vi "New Image.vi"(8 "error in (no error)":errorcluster, 9 "Height":i32, 10 "Width":i32) -> (0 "error out":errorcluster, 3 "Image out":refnum<class "Image.lvclass">)   [LabVIEW 2020, in "RPI.SenseHat.Display.lvlib" / "Image.lvclass"]
uses:
  Image.lvclass
  Pixel/Pixel.lvclass
  Color/Color.lvclass
  Image.lvclass/Image.ctl
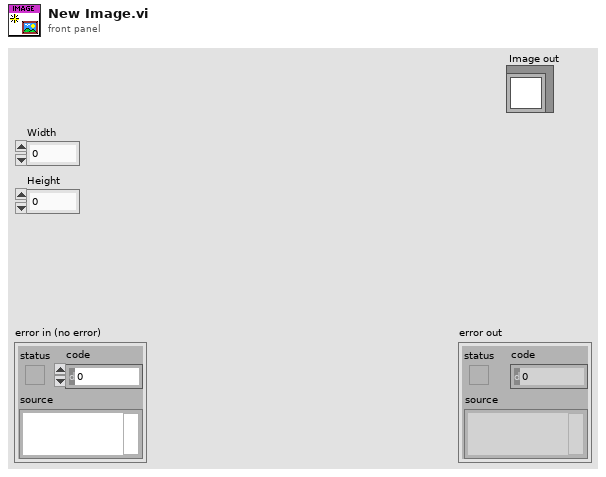
[diagram p1: front panel]
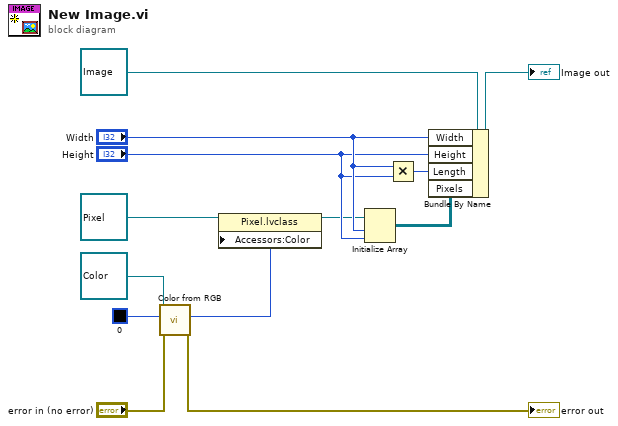
[diagram p0: block diagram]
diagram:
  n1 = call "Color from RGB.vi"("error in (no error)"="error in (no error)", "Color Box"=u32 0, "Color in"=refnum<class "Color.lvclass"> refnum) -> ("error out"=→"error out":errorcluster, "Color"=w1:u16)  [unwired: 6 in, 1 out]
  n2 = property class="Pixel.lvclass"(reference=refnum<class "Pixel.lvclass"> refnum ("Pixel.lvclass"), "Accessors:Color"=w1) -> (reference out=w2:refnum<class "Pixel.lvclass">)  [unwired: 1 in, 1 out]
  n3 = Initialize Array(w2, "Width", "Height") -> (w8:refnum<class "Pixel.lvclass">[][])
  n4 = Multiply(x="Width", y="Height") -> (x*y=w11:i32)
  n5 = Bundle By Name(cluster=refnum<class "Image.lvclass"> refnum ("Image in"), "Width"="Width", "Height"="Height", "Length"=w11, "Pixels"=w8) -> (→"Image out":refnum<class "Image.lvclass">)
